vi "DBSqlSelectToArray(2DArrayString).vi"(6 "String":string, 7 "shift reg in":string[][](array[string]), 9 "enable":bool, 10 "format":string[][](array[string]), 11 "connection information":path) -> (0 "error out":errorcluster, 3 "shift reg out":string[][](array[string]))   [LabVIEW 2011]
uses:
  <vilib>/addons/database/Connection.llb/DB Tools Open Connec (Path).vi
  <vilib>/addons/database/Connection.llb/Conn Execute.vi
  <vilib>/addons/database/Recordset.llb/Rec Fetch Recordset Data (R).vi
  <vilib>/addons/database/Recordset.llb/Rec Destroy - Connection.vi
  <vilib>/addons/database/_DB Variant To Data/Database Variant To Data.xnode
  <vilib>/addons/database/NI_Database_API.lvlib
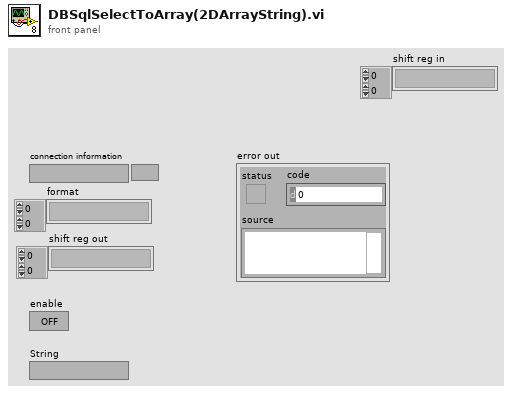
[diagram p1: front panel]
types:
  T1 = typedef "NI_Database_API.lvlib/Conn ObjectReference.ctl" = refnum<k1>
  T2 = typedef "NI_Database_API.lvlib/Rec ObjectReference.ctl" = refnum<k1>
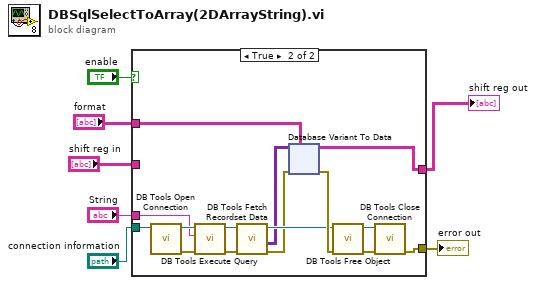
[diagram p0: block diagram]
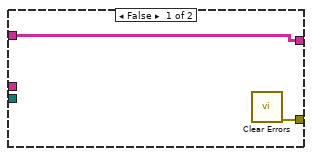
[diagram p2: hidden frame]
diagram:
  n1 = case shown="True" "enable" {
    tunnel: [w8 w14] -> w2
    tunnel: "String" -> [_ w13]
    tunnel: [w9 w12] -> w5
    tunnel: "connection information" -> [_ w11]
    tunnel: "format" -> [_ w10]
    tunnel: "shift reg in" -> [w8 _]
    frame False {
      n2 = call <vilib>:"Clear Errors.vi"() -> ("error out"=w9:errorcluster)  [unwired: 7 in]
    }
    frame True {
      n3 = call-poly <vilib>:"DB Tools Open Connection.vi"("connection information"=w11) -> ("error out"=w19:errorcluster, "connection reference"=w20:T1)  [unwired: 7 in]
      n4 = call-poly <vilib>:"DB Tools Execute Query.vi"("error in (no error)"=w19, "SQL query"=w13, "connection reference"=w20) -> ("error out"=w16:errorcluster, "recordset reference"=w15:T2)  [unwired: 5 in]
      n5 = call-poly <vilib>:"DB Tools Fetch Recordset Data.vi"("error in (no error)"=w16, "recordset reference"=w15) -> ("error out"=w17:errorcluster, "recordset data"=w18:variant[][], "recordset reference out"=w21:T2)  [unwired: 3 in]
      n6 = xnode "Database Variant To Data"("database variant"=w18, "error in"=w17, "type"=w10) -> ("data"=w14:string[][], "error out"=w23:errorcluster)
      n7 = call-poly <vilib>:"DB Tools Free Object.vi"("error in (no error)"=w23, "recordset reference"=w21) -> ("error out"=w24:errorcluster, "connection reference"=w22:T1)  [unwired: 8 in]
      n8 = call <vilib>:"DB Tools Close Connection.vi"("error in (no error)"=w24, "connection reference"=w22) -> ("error out"=w12:errorcluster)  [unwired: 5 in]
    }
  }
  "error out" <- w5
  "shift reg out" <- w2
